vi "Gradient BG Color.vi"(6 "Row Or Col":T1, 8 "错误输入":errorcluster, 9 "End":u32(colorbox), 10 "Start":u32(colorbox), 11 "Mlistbox Ref":refnum<vi>) -> (0 "错误输出":errorcluster, 3 "Mlistbox Ref Dup":refnum<vi>)   [LabVIEW 2012, in "Mlistbox Tools.lvlib"]
uses:
  Mlistbox Tools.lvlib
  Custom Type/Row and Col Option.ctl
  ListBox/Custom Type/Read and Write Mode.ctl
  Property/Set and Get Num of Rows Or Cols.vi
  Property/Set and Get Active Cell BG Color.vi
  ListBox/Listbox Tool.lvlib
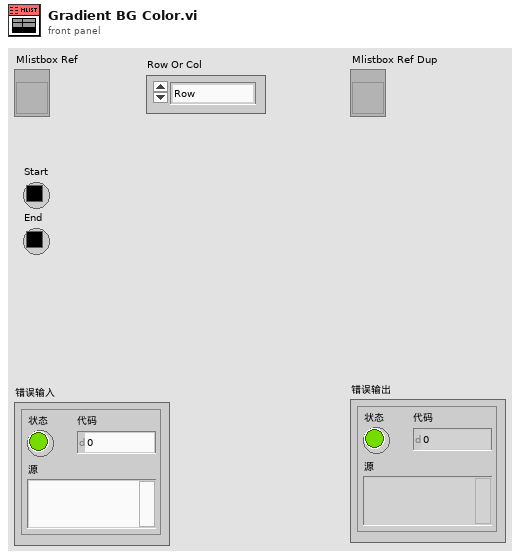
[diagram p1: front panel]
types:
  T1 = typedef "Mlistbox Tools.lvlib/Row and Col Option.ctl" = enum16{"Row", "Col"}
  T2 = typedef "Listbox Tool.lvlib/Read and Write Mode.ctl" = enum16{"Read", "Write"}
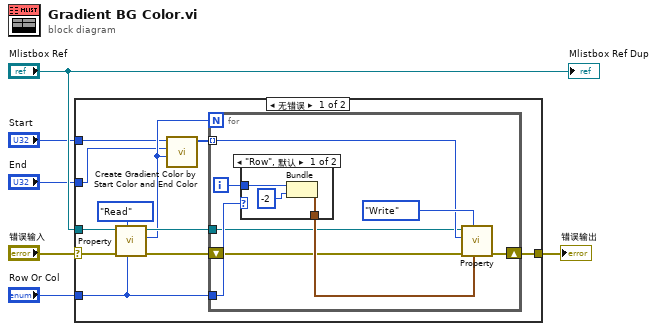
[diagram p0: block diagram]
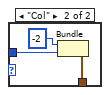
[diagram p2: hidden frame]
diagram:
  n1 = case shown="无错误" "错误输入" {
    selector: "错误输入" -> [w13 w32]
    tunnel: "Row Or Col" -> [w17 _]
    tunnel: [w12 w32] -> w4
    tunnel: "Mlistbox Ref" -> [w16 _]
    tunnel: "Start" -> [w9 _]
    tunnel: "End" -> [w8 _]
    frame No Error {
      n2 = call-poly "Property.vi"("Row Or Col"=w17, "Mode"=Read_and_Write_Mode."Read", "错误输入"=w13, "Mlistbox Ref"=w16) -> ("错误输出"=w11:errorcluster, "Number of Rows or Cols Out"=w10:u32, "Mlistbox Ref Dup"=w14:refnum<vi>)  [unwired: 5 in]
      n3 = call "Create Gradient Color by Start Color and End Color.vi"("Length"=w10, "End"=w8, "Start"=w9) -> ("ColorArray"=w7:u32[])  [unwired: 7 in, 1 out]
      n4 = for {
        N: w10 -> [_]
        tunnel: w17 -> [w25]
        tunnel: w14 -> [w19]
        shift-right: [w24] -> w12
        shift-left: w11 -> [w18]
        tunnel: w7 -> [w21] mode=indexing
        i -> [w22]
        n5 = case shown="\"Row\", 默认" w25 {
          tunnel: w22 -> [w28 w31]
          tunnel: [w26 w29] -> w20
          frame "Row", Default {
            n6 = Bundle(w28, -2) -> (w26:cluster{i32, i32})  [unwired: 1 in]
          }
          frame "Col" {
            n7 = Bundle(-2, w31) -> (w29:cluster{i32, i32})  [unwired: 1 in]
          }
        }
        n8 = call-poly "Property.vi"("Active Cell In"=w20, "Mode"=Read_and_Write_Mode."Write", "错误输入"=w18, "Active Cell BG Color In"=w21, "Mlistbox Ref"=w19) -> ("错误输出"=w24:errorcluster)  [unwired: 4 in, 2 out]
      }
    }
    frame Error {
    }
  }
  "错误输出" <- w4
  "Mlistbox Ref Dup" <- "Mlistbox Ref"
